vi "Spawn Eldest.vi"(9 "UID":string, 10 "Actor":refnum<class "Actor.lvclass">) -> (0 "Error out":errorcluster, 5 "Actor out":refnum<class "Actor.lvclass">)   [LabVIEW 2025, in "jettl.lvlib" / "Actor.lvlib"]
uses:
  Actor.lvlib
  Actor/Actor.lvclass
  Base Actor/Base Actor.lvclass
  C:/git/jettl/src/jettl/jettl/Actor/Actor/Actor.lvclass
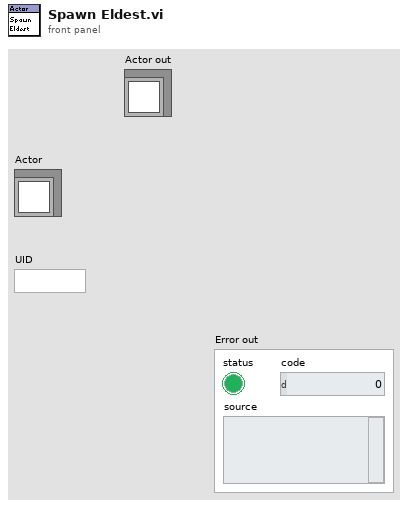
[diagram p1: front panel]
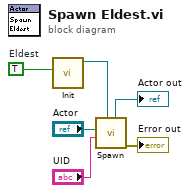
[diagram p0: block diagram]
diagram:
  w3 = TRUE  # Eldest
  n1 = call "Init.vi"("Eldest"=w3) -> ("Base Actor out"=w4:refnum<class "Base Actor.lvclass">)  [unwired: 10 in]
  n2 = call "Spawn.vi"("Actor in"=w4, "UID"="UID", "Actor"="Actor") -> ("Error out"=→"Error out":errorcluster, "Actor out"=→"Actor out":refnum<class "Base Actor.lvclass">)  [unwired: 7 in]
